vi "ExFileReadNDisplayGbl.vi"() -> ()   [LabVIEW 2010]
panel:
  in  "Quick Select":u32(knob) min=1 max=1000 scale=1.0..99.0
  in  "Set Position":bool
  in  "Image Number":u32=1 min=1 step=1
  in  "Timeout":i32=-1
  out "First Time Flag":bool=TRUE
  out "Update Flag":bool
  in  "Ending":bool
  in  "Beginning":bool
  out "Frame Number":i32
  in  "Backward":bool
  in  "Forward":bool
  in  "Full File Name":path
  in  "Stop":bool
  in  "FileType":u32=67174400
  out "error out":errorcluster
  in  "error in (no error)":errorcluster
  # "ExReadFileNDisplayGbl.vi\nThis example will read in a file of the\nselected data type and display all frames.\nWhen finished viewing data, make sure to\nuse the STOP button to close the display."
  # "File Types:\nSPE = 67371008\nTIF   = 67174400\nPMI  = 67436544"
  # "NOTICE\nTHIS VI REQUIRES THAT THE TOOLKIT BE UNLOADED BY RUNNING THE  VI EXCLOSEGLOBALCAM.VI\n BEFORE LEAVING LABVIEW."
  # "Browse match pattern is set to *.tif.  Modify this if different file type is needed."
  # "This will properly close\nthe image and\ndeallocate memory."
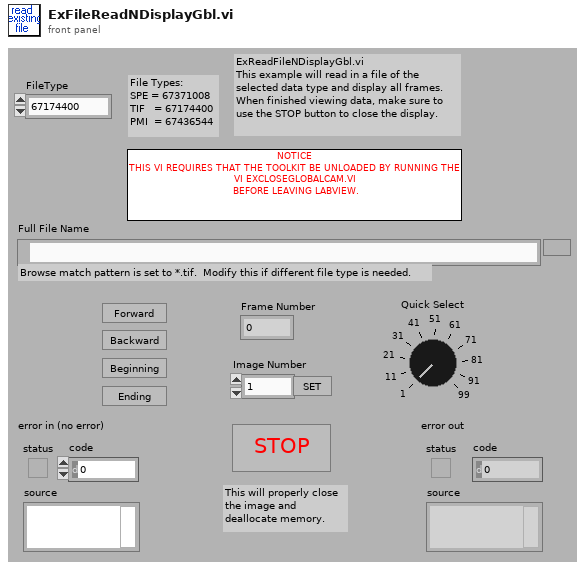
[diagram p1: front panel]
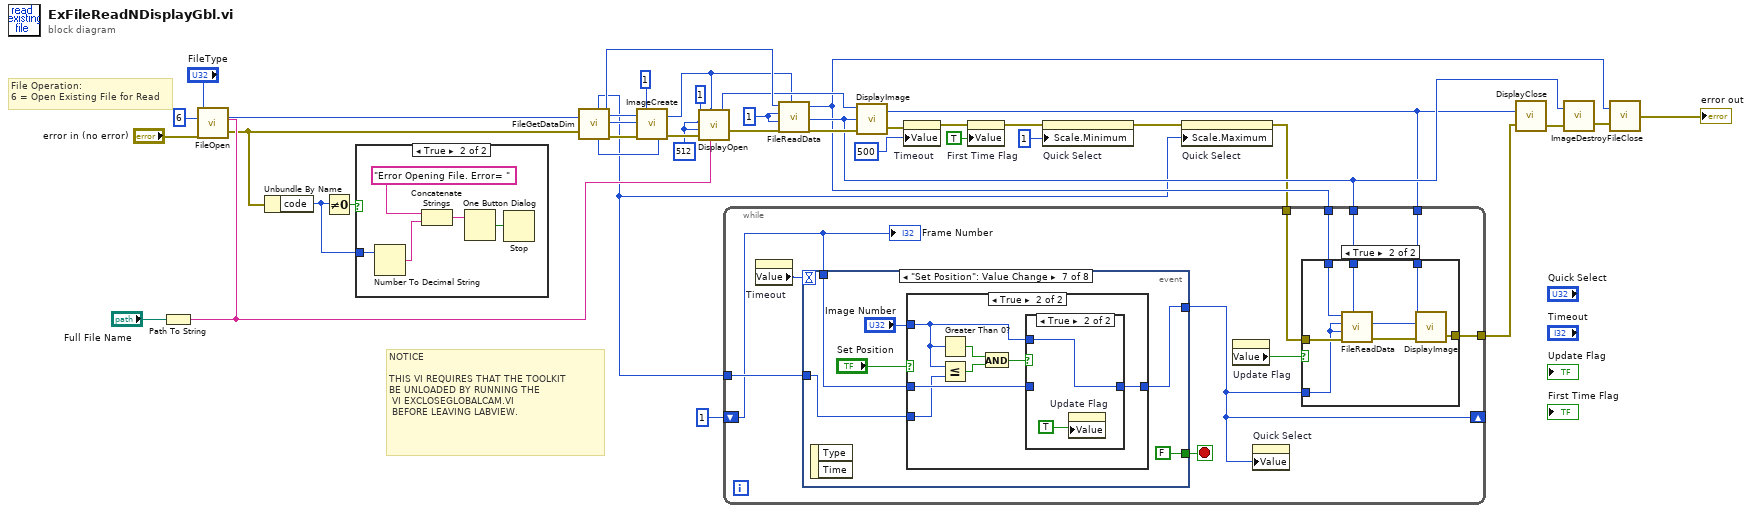
[diagram p0: block diagram]
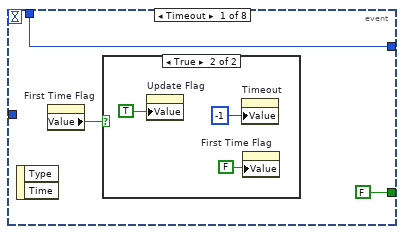
[diagram p3: hidden frame]
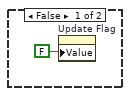
[diagram p4: hidden frame]
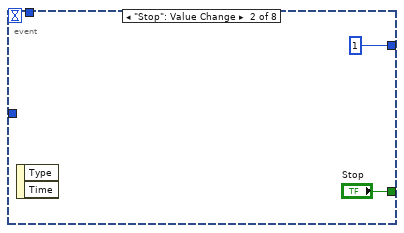
[diagram p5: hidden frame]
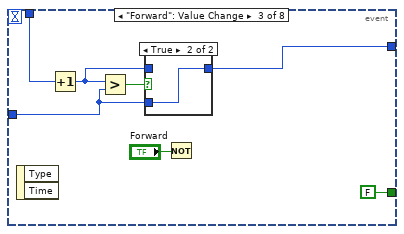
[diagram p6: hidden frame]
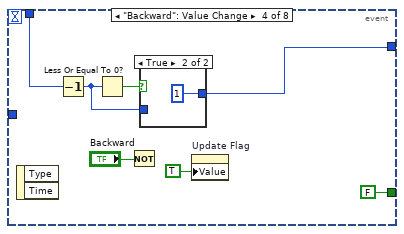
[diagram p8: hidden frame]
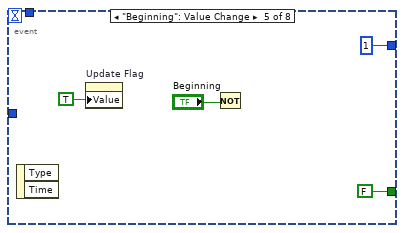
[diagram p10: hidden frame]
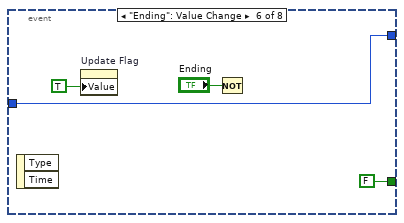
[diagram p11: hidden frame]
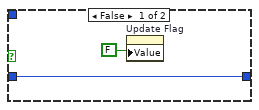
[diagram p12: hidden frame]
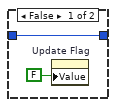
[diagram p13: hidden frame]
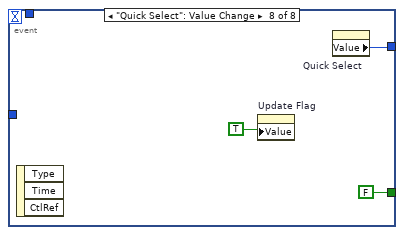
[diagram p14: hidden frame]
diagram:
  w22 = 1
  w31 = 512
  # "NOTICE\n\nTHIS VI REQUIRES THAT THE TOOLKIT\nBE UNLOADED BY RUNNING THE\n VI EXCLOSEGLOBALCAM.VI\n BEFORE LEAVING LABVIEW."
  # "File Operation:\n6 = Open Existing File for Read"
  n1 = Path To String(path="Full File Name") -> (string=w26:string)
  n2 = call <userlib>:"FileOpen.vi"("error in"="error in (no error)", "File Operations"=u32 6 ("File Operation"), "FileName"=w26, "File Type"="FileType") -> ("error out"=w6:errorcluster, "File Handle"=w17:u32)
  n3 = Unbundle By Name(w6) -> ("code"=w7:i32)
  n4 = Not Equal To 0?(x=w7) -> (x != 0?=w8:bool)
  n5 = case shown="True" w8 {
    tunnel: w7 -> [_ w41]
    frame False {
    }
    frame True {
      n6 = Number To Decimal String(number=w41) -> (decimal integer string=w42:string)  [unwired: 1 in]
      n7 = Concatenate Strings("Error Opening File. Error= ", w42) -> (w44:string)
      n8 = One Button Dialog(message=w44) -> (true=w43:bool)  [unwired: 1 in]
      n9 = Stop(stop? (T)=w43) -> ()
    }
  }
  n10 = call <userlib>:"FileGetDataDim.vi"("File Handle"=w17, "error in"=w6) -> ("Number of Frames"=w1:u32, "Data Type"=w34:u32, "File Handle"=w21:u32, "X dim"=w36:u32, "Y dim"=w35:u32, "error out"=w37:errorcluster)
  n11 = call <userlib>:"ImageCreate.vi"("X dimension"=w36, "Y dimension"=w35, "Data Type"=w34, "error in"=w37, "Number Of Frames"=1) -> ("Image Handle"=w18:u32, "error out"=w33:errorcluster)
  n12 = call <userlib>:"DisplayOpen.vi"("Display Title"=w26, "Image Handle"=w18, "error in"=w33, "Display Height"=w31, "Display Width"=w31, "Display Type"=1) -> ("error out"=w23:errorcluster, "Display Handle"=w19:u32)
  n13 = call <userlib>:"FileReadData.vi"("File Handle"=w21, "Start Frame"=w22, "End Frame"=w22, "error in"=w23, "Image Handle"=w18) -> ("File Handle"=w9:u32, "Image Handle"=w15:u32, "error out"=w20:errorcluster)
  n14 = call <userlib>:"DisplayImage.vi"("error in"=w20, "Image Handle"=w15, "Display Handle"=w19) -> ("error out"=w14:errorcluster, "Display Handle"=w10:u32)  [unwired: 1 in]
  n15 = property on="Timeout" class="DigNum (strict)"(error in=w14, "Value"=500) -> (error out=w12:errorcluster)  [unwired: 1 in, 1 out]
  n16 = property on="First Time Flag" class="Bool (strict)"(error in=w12, "Value"=TRUE) -> (error out=w5:errorcluster)  [unwired: 1 in, 1 out]
  n17 = property on="Quick Select" class="Knob (strict)"(error in=w5, "Scale.Minimum"=1) -> (error out=w4:errorcluster)  [unwired: 1 in, 1 out]
  n18 = property on="Quick Select" class="Knob (strict)"(error in=w4, "Scale.Maximum"=w1) -> (error out=w3:errorcluster)  [unwired: 1 in, 1 out]
  n19 = while {
    shift-right: [w46] -> _
    shift-left: 1 -> [w50]
    tunnel: w9 -> [w56]
    tunnel: w15 -> [w55]
    tunnel: w10 -> [w54]
    tunnel: [w53] -> w16
    tunnel: w1 -> [w51]
    tunnel: w3 -> [w47]
    stop <- w49 stop-if-true
    n20 = property on="Timeout" class="DigNum (strict)"() -> ("Value"=w52:i32)  [unwired: 2 in, 2 out]
    n21 = event shown="[6] \"Set Position\": Value Change" {
      selector: _ -> [_ _ _ _ _ _ _ _]
      dyn-events: _ -> [_ _ _ _ _ _ _ _]
      timeout: w52 -> [_ _ _ _ _ _ _ _]
      tunnel: w50 -> [w58 _ w70 w79 _ _ w95 _]
      tunnel: w51 -> [_ _ w69 _ _ w88 w94 _]
      tunnel: [w58 1 w68 w75 1 w88 w93 w113] -> w46
      tunnel: [FALSE "Stop" FALSE FALSE FALSE FALSE FALSE FALSE] -> w49
      event Timeout {
        n22 = event-data() -> ()  [unwired: 1 in, 2 out]
        n23 = property on="First Time Flag" class="Bool (strict)"() -> ("Value"=w59:bool)  [unwired: 2 in, 2 out]
        n24 = case shown="True" w59 {
          frame False {
            n25 = property on="Update Flag" class="Bool (strict)"("Value"=FALSE) -> ()  [unwired: 2 in, 2 out]
          }
          frame True {
            n26 = property on="Update Flag" class="Bool (strict)"("Value"=TRUE) -> ()  [unwired: 2 in, 2 out]
            n27 = property on="Timeout" class="DigNum (strict)"("Value"=-1) -> ()  [unwired: 2 in, 2 out]
            n28 = property on="First Time Flag" class="Bool (strict)"("Value"=FALSE) -> ()  [unwired: 2 in, 2 out]
          }
        }
      }
      event "Stop": Value Change {
        n29 = event-data() -> ()  [unwired: 1 in, 2 out]
      }
      event "Forward": Value Change {
        n30 = event-data() -> ()  [unwired: 1 in, 2 out]
        n31 = Increment(x=w70) -> (x+1=w72:u32)
        n32 = Greater?(x=w72, y=w69) -> (0:w71:bool)
        n33 = case shown="True" w71 {
          tunnel: w69 -> [_ w74]
          tunnel: [w73 w74] -> w68
          tunnel: w72 -> [w73 _]
          frame False {
          }
          frame True {
          }
        }
        n34 = Not(x="Forward") -> ()  [unwired: 1 out]
      }
      event "Backward": Value Change {
        n35 = event-data() -> ()  [unwired: 1 in, 2 out]
        n36 = Decrement(x=w79) -> (x-1=w81:u32)
        n37 = Less Or Equal To 0?(x=w81) -> (x <= 0?=w80:bool)
        n38 = Not(x="Backward") -> ()  [unwired: 1 out]
        n39 = case shown="True" w80 {
          tunnel: [w82 1] -> w75
          tunnel: w81 -> [w82 _]
          frame False {
          }
          frame True {
          }
        }
        n40 = property on="Update Flag" class="Bool (strict)"("Value"=TRUE) -> ()  [unwired: 2 in, 2 out]
      }
      event "Beginning": Value Change {
        n41 = event-data() -> ()  [unwired: 1 in, 2 out]
        n42 = property on="Update Flag" class="Bool (strict)"("Value"=TRUE) -> ()  [unwired: 2 in, 2 out]
        n43 = Not(x="Beginning") -> ()  [unwired: 1 out]
      }
      event "Ending": Value Change {
        n44 = event-data() -> ()  [unwired: 1 in, 2 out]
        n45 = property on="Update Flag" class="Bool (strict)"("Value"=TRUE) -> ()  [unwired: 2 in, 2 out]
        n46 = Not(x="Ending") -> ()  [unwired: 1 out]
      }
      event "Set Position": Value Change {
        n47 = event-data() -> ()  [unwired: 1 in, 2 out]
        n48 = case shown="True" "Set Position" {
          tunnel: w95 -> [w99 w101]
          tunnel: [w99 w102] -> w93
          tunnel: "Image Number" -> [_ w103]
          tunnel: w94 -> [_ w100]
          frame False {
            n49 = property on="Update Flag" class="Bool (strict)"("Value"=FALSE) -> ()  [unwired: 2 in, 2 out]
          }
          frame True {
            n50 = Greater Than 0?(x=w103) -> (x > 0?=w105:bool)
            n51 = Less Or Equal?(x=w103, y=w100) -> (x <= y?=w104:bool)
            n52 = And(x=w105, y=w104) -> (x .and. y?=w106:bool)
            n53 = case shown="True" w106 {
              tunnel: w103 -> [_ w110]
              tunnel: [w108 w110] -> w102
              tunnel: w101 -> [w108 _]
              frame False {
                n54 = property on="Update Flag" class="Bool (strict)"("Value"=FALSE) -> ()  [unwired: 2 in, 2 out]
              }
              frame True {
                n55 = property on="Update Flag" class="Bool (strict)"("Value"=TRUE) -> ()  [unwired: 2 in, 2 out]
              }
            }
          }
        }
      }
      event "Quick Select": Value Change {
        n56 = event-data() -> ()  [unwired: 1 in, 3 out]
        n57 = property on="Update Flag" class="Bool (strict)"("Value"=TRUE) -> ()  [unwired: 2 in, 2 out]
        n58 = property on="Quick Select" class="Knob (strict)"() -> ("Value"=w113:u32)  [unwired: 2 in, 2 out]
      }
    }
    n59 = property on="Update Flag" class="Bool (strict)"() -> ("Value"=w48:bool)  [unwired: 2 in, 2 out]
    n60 = property on="Quick Select" class="Knob (strict)"("Value"=w46) -> ()  [unwired: 2 in, 2 out]
    n61 = case shown="True" w48 {
      tunnel: w46 -> [_ w116]
      tunnel: w47 -> [w114 w120]
      tunnel: w56 -> [_ w119]
      tunnel: w55 -> [_ w118]
      tunnel: w54 -> [_ w115]
      tunnel: [w114 w117] -> w53
      frame False {
      }
      frame True {
        n62 = call <userlib>:"FileReadData.vi"("File Handle"=w119, "Start Frame"=w116, "End Frame"=w116, "error in"=w120, "Image Handle"=w118) -> ("Image Handle"=w121:u32, "error out"=w122:errorcluster)  [unwired: 1 out]
        n63 = call <userlib>:"DisplayImage.vi"("error in"=w122, "Image Handle"=w121, "Display Handle"=w115) -> ("error out"=w117:errorcluster)  [unwired: 1 in, 1 out]
      }
    }
    "Frame Number" <- w50
  }
  n64 = call <userlib>:"DisplayClose.vi"("error in"=w16, "Display Handle"=w10) -> ("error out"=w29:errorcluster)
  n65 = call <userlib>:"ImageDestroy.vi"("error in"=w29, "Data handle"=w15) -> ("error out"=w28:errorcluster)
  n66 = call <userlib>:"FileClose.vi"("error in"=w28, "File Handle"=w9) -> ("error out"=→"error out":errorcluster)
